vi "CRY6181 Run Seq.vi"() -> ()   [LabVIEW 2013]
uses:
  CRYSystem/Typedef Control/CRYData Cluster.ctl
  CRYSystem/Typedef Control/CRYResult Cluster.ctl
  CRYSystem/Typedef Control/CRYWaveform Cluster.ctl
  CRYWindow/SubVI/CRYMain Sub Window Global.vi
  CRYProject/CRYProject Editor Global.vi
  CRYMainGlobal.vi
  CRYSystem/Task Sequence/CRYProject Run Control Global.vi
panel:
  in  "Tab Control":enum32{"Parameter", "Data"}(tab)
  out "Margin":dbl
  out "Duration":dbl
  out "Passed?":bool
  out "Ran to completion":bool
  in  "path":path caption="Sequence to run (full path)"
  in  "Serial #":string
  in  "Lot #":string
  in  "Mode":enum16{"Load Sequence", "Run Sequence", "All"}(ring)
  out "Data Array":T1[](array[typedef]) {"Z data" items=["dB", "Lin"]; "X data" items=["dB", "Lin"]; "Y data" items=["dB", "Lin"]; "Z dB ref" format="%.1f"; "Z axis" items=["Log", "Lin"]; "X dB ref" format="%.1f"; "X axis" items=["Log", "Lin"]; "Y axis" items=["Log", "Lin"]; "Y dB ref" format="%.1f"; "Curve"."z" format="%.2f"; "Curve"."y" format="%.2f"; "Curve"."x" format="%.2f"}
  out "Results Array":T2[](array[typedef]) {"Margin" format="%.2f"}
  out "Waveforms Array":T3[](array[typedef]) {"Y dB ref" format="%.1f"; "Y axis" items=["Log", "Lin"]; "Y data" items=["dB", "Lin"]; "X data" items=["dB", "Lin"]}
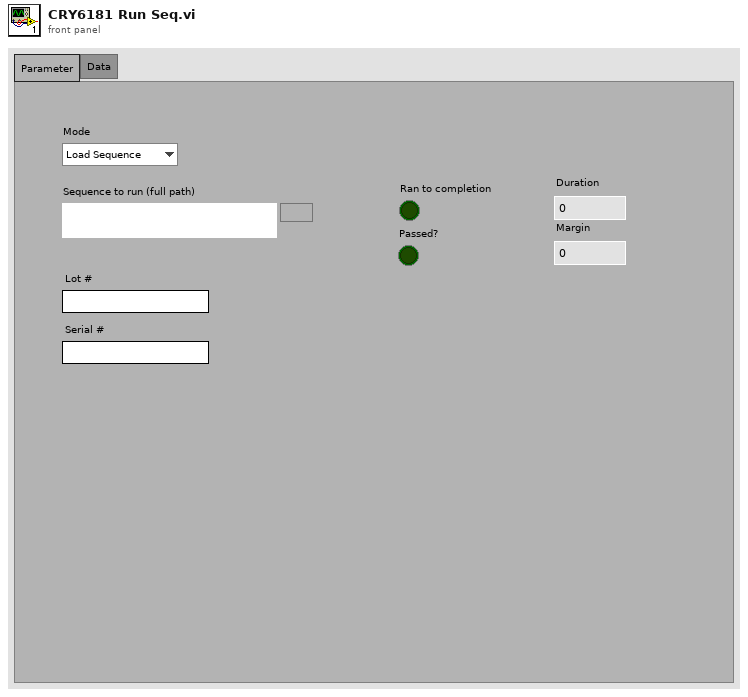
[diagram p1: front panel]
types:
  T1 = typedef "CRYData Cluster.ctl" = cluster{"Name":string, "Curve":cluster{"x":dbl, "y":dbl, "z":dbl}[], "X data":u16, "Y data":u16, "Z data":u16, "X axis":u16, "Y axis":u16, "Z axis":u16, "X unit":string, "Y unit":string, "Z unit":string, "X dB ref":dbl, "Y dB ref":dbl, "Z dB ref":dbl, "single val":bool, "protected":bool, "display X":bool, "display Y":bool, "display Z":bool, "Test Info":string, "Step No.":i32, "Plot Settings":cluster{"Color":u32, "Interpolation":u8, "Point Style":u8, "Line Style":u8, "Point Color":u32, "Line Width":u8, "Bar Plot Style":u8, "Fill To":i16}, "AutoProtect":bool}
  T2 = typedef "CRYResult Cluster.ctl" = cluster{"Name":string, "Margin":dbl, "unit":string, "Verdict":bool, "Limit":string, "Max/Min":string, "protected":bool, "Step No.":i32, "Test Info":string, "AutoProtect":bool}
  T3 = typedef "CRYWaveform Cluster.ctl" = cluster{"Waveform":cluster{"X0":dbl, "dX":dbl, "Y":sgl[]}, "X data":u16, "Y data":u16, "Y axis":u16, "X unit":string, "Y unit":string, "Y dB ref":dbl, "display Y":bool, "display X":bool, "Overload?":bool, "Test Info":string, "Step No.":i32, "Name":string, "protected":bool, "Sqc history":string[], "Signal Channel ID":i32, "Plot Settings":cluster{"Color":u32, "Interpolation":u8, "Point Style":u8, "Line Style":u8, "Point Color":u32, "Line Width":u8, "Bar Plot Style":u8, "Fill To":i16}, "AutoProtect":bool}
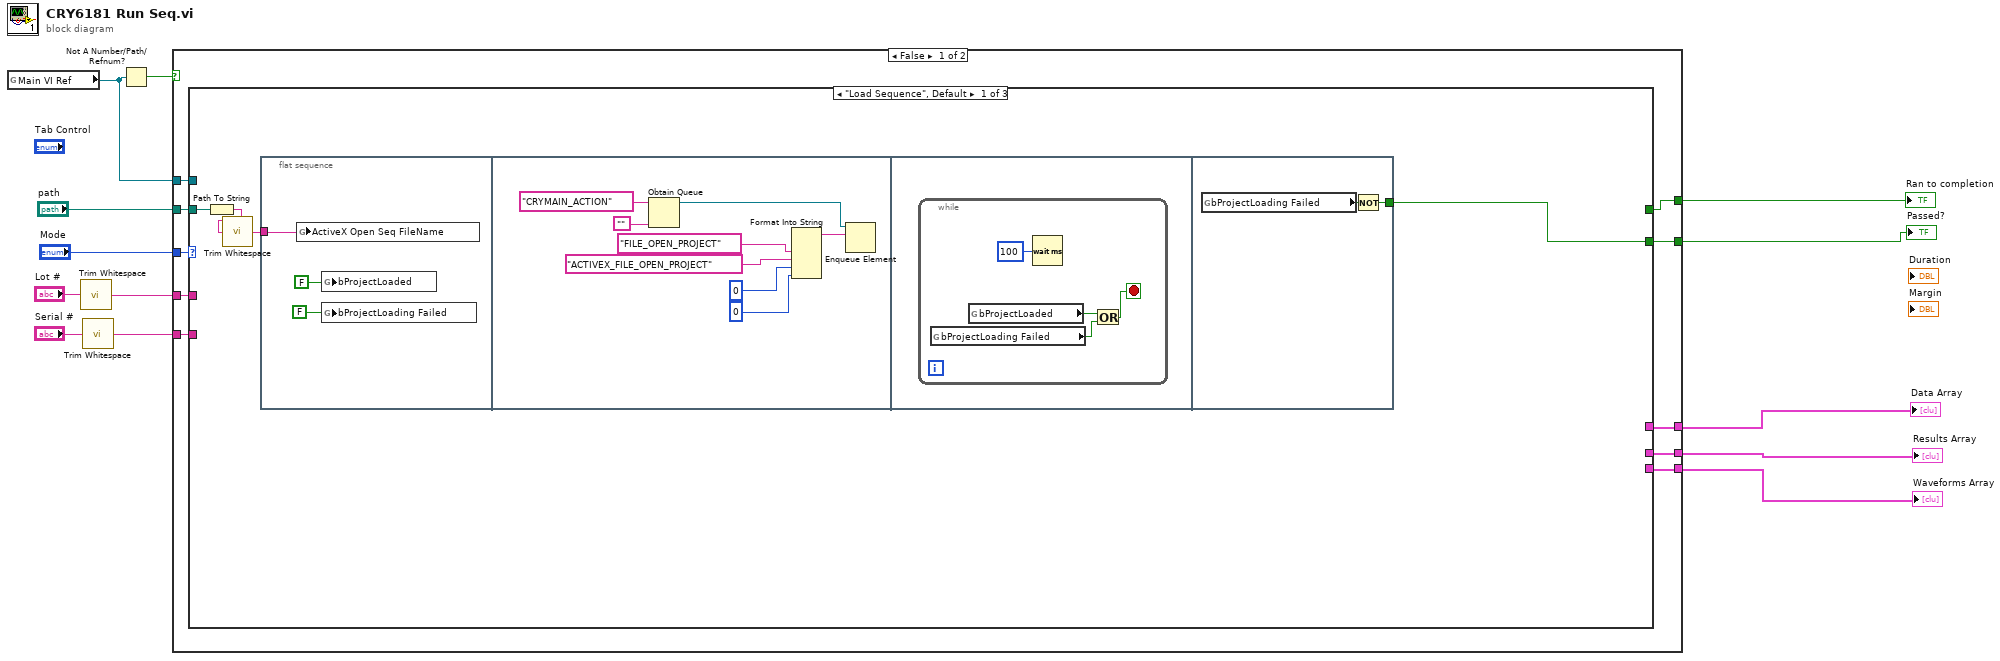
[diagram p0: block diagram]
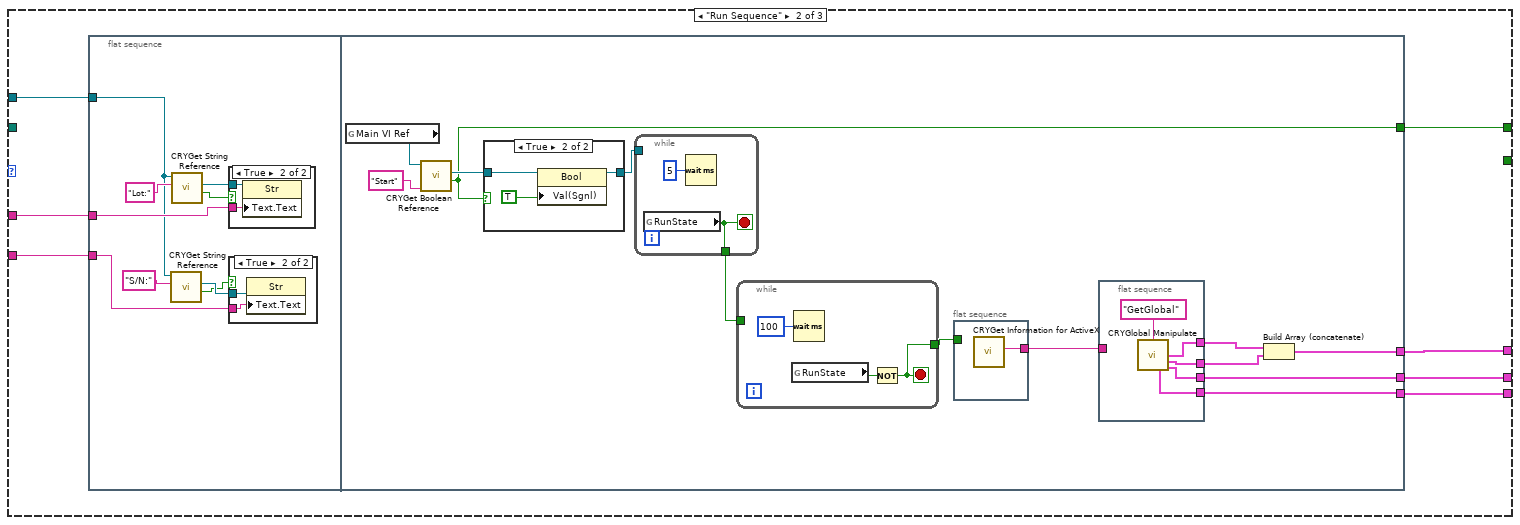
[diagram p2: hidden frame]
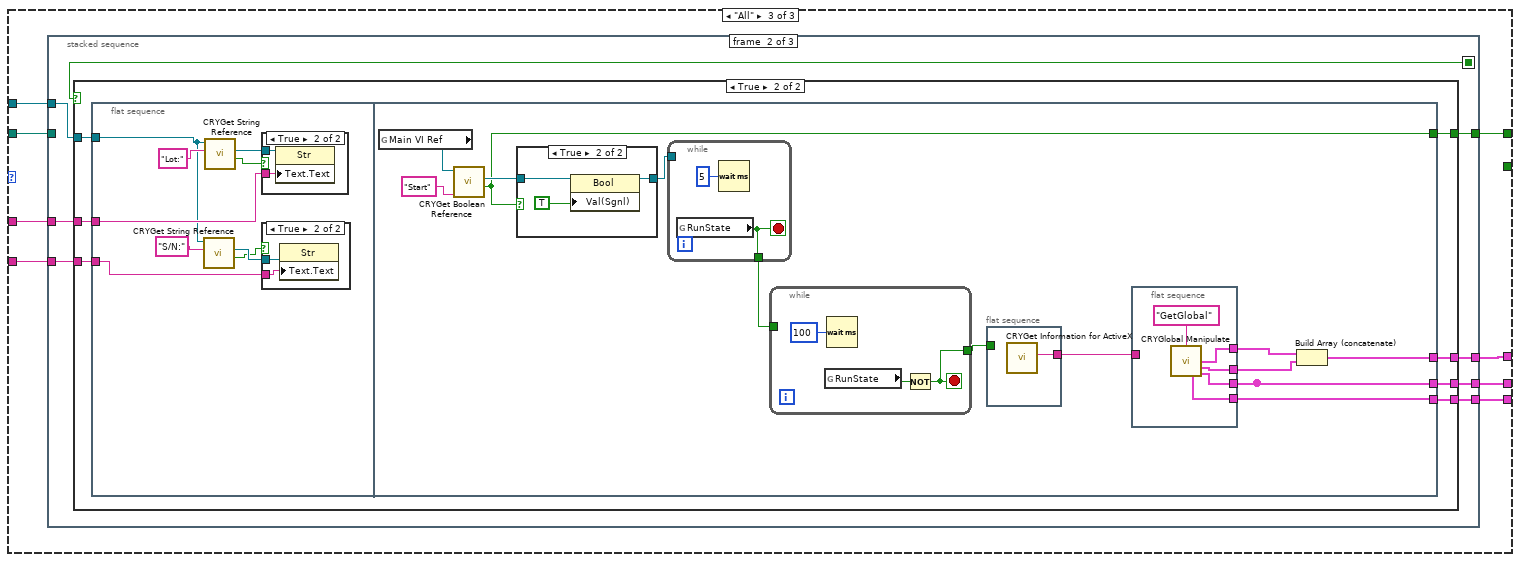
[diagram p6: hidden frame]
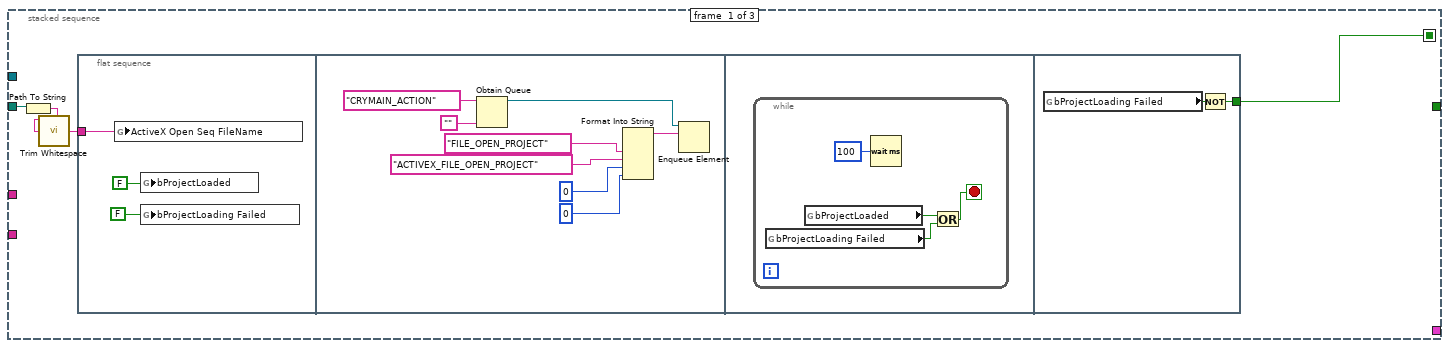
[diagram p7: hidden frame]
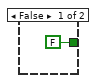
[diagram p8: hidden frame]
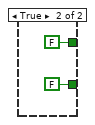
[diagram p13: hidden frame]
diagram:
  n1 = global read "CRYMain Sub Window Global.vi" "Main VI Ref"() -> (w1:refnum<vi>)
  n2 = call <vilib>:"Trim Whitespace.vi"("string"="Lot #") -> ("trimmed string"=w11:string)  [unwired: 1 in]
  n3 = call <vilib>:"Trim Whitespace.vi"("string"="Serial #") -> ("trimmed string"=w9:string)  [unwired: 1 in]
  n4 = Not A Number/Path/Refnum?(number/path/refnum=w1) -> (NaN/Path/Refnum?=w2:bool)
  n5 = case shown="False" w2 {
    tunnel: "Mode" -> [w23 _]
    tunnel: w11 -> [w22 _]
    tunnel: w9 -> [w21 _]
    tunnel: [w20 FALSE ("Exist?")] -> w8
    tunnel: [w19 _] -> w7
    tunnel: [w18 _] -> w6
    tunnel: [w17 _] -> w5
    tunnel: "path" -> [w16 _]
    tunnel: [w15 FALSE] -> w3
    tunnel: w1 -> [w14 _]
    frame False {
      n6 = case shown="\"Load Sequence\", Default" w23 {
        tunnel: w22 -> [_ w51 w99]
        tunnel: w21 -> [_ w50 w98]
        tunnel: [_ w49 w94] -> w20
        tunnel: [_ w48 w97] -> w19
        tunnel: [_ w47 w96] -> w18
        tunnel: [_ w46 w95] -> w17
        tunnel: w16 -> [w27 _ w100]
        tunnel: [w24 _ _] -> w15
        tunnel: w14 -> [_ w45 w93]
        frame "Load Sequence", Default {
          n7 = Path To String(path=w27) -> (string=w25:string)
          n8 = call <vilib>:"Trim Whitespace.vi"("string"=w25) -> ("trimmed string"=w26:string)  [unwired: 1 in]
          n9 = flat-sequence {
            tunnel: w26 -> [w30]
            tunnel: [w43] -> w24
            frame #0 {
              n10 = global write "CRYMainGlobal.vi" "ActiveX Open Seq FileName"(w30) -> ()
              n11 = global write "CRYProject Editor Global.vi" "bProjectLoaded"(FALSE (".not. x?")) -> ()
              n12 = global write "CRYProject Editor Global.vi" "bProjectLoading Failed"(FALSE ("bProjectLoaded Failed")) -> ()
            }
            frame #1 {
              n13 = Obtain Queue(name (unnamed)="CRYMAIN_ACTION" ("YAxisTitle"), element data type="" ("Action Type")) -> (queue out=w32:refnum<queue>)  [unwired: 3 in, 2 out]
              n14 = Format Into String("FILE_OPEN_PROJECT" ("input 1"), "ACTIVEX_FILE_OPEN_PROJECT" ("input 2"), 0 ("input 2"), 0 ("input 3")) -> (resulting string=w37:string)  [unwired: 3 in, 1 out]
              n15 = Enqueue Element(queue=w32, element=w37) -> ()  [unwired: 1 in, 4 out]
            }
            frame #2 {
              n16 = while {
                stop <- w39 stop-if-true
                n17 = global read "CRYProject Editor Global.vi" "bProjectLoading Failed"() -> (w40:bool)
                n18 = global read "CRYProject Editor Global.vi" "bProjectLoaded"() -> (w41:bool)
                n19 = Wait (ms)(milliseconds to wait=u32 100) -> ()  [unwired: 1 out]
                n20 = Or(x=w41, y=w40) -> (x .or. y?=w39:bool)
              }
            }
            frame #3 {
              n21 = global read "CRYProject Editor Global.vi" "bProjectLoading Failed"() -> (w44:bool)
              n22 = Not(x=w44) -> (.not. x?=w43:bool)
            }
          }
        }
        frame "Run Sequence" {
          n23 = flat-sequence {
            tunnel: w51 -> [w57]
            tunnel: w50 -> [w54]
            tunnel: w45 -> [w52]
            tunnel: [w71] -> w49
            tunnel: [w67] -> w48
            tunnel: [w66] -> w46
            tunnel: [w65] -> w47
            frame #0 {
              n24 = call "CRYGet String Reference.vi"("Label Name"="S/N:", "VI Refnum"=w52) -> ("Find?"=w53:bool, "String Ref Out"=w55:refnum<vi>)  [unwired: 7 in, 1 out]
              n25 = call "CRYGet String Reference.vi"("Label Name"="Lot:", "VI Refnum"=w52) -> ("Find?"=w58:bool, "String Ref Out"=w59:refnum<vi>)  [unwired: 7 in, 1 out]
              n26 = case shown="True" w58 {
                tunnel: w59 -> [_ w64]
                tunnel: w57 -> [_ w63]
                frame False {
                }
                frame True {
                  n27 = property class="Str"(reference=w64, "Text.Text"=w63) -> ()  [unwired: 1 in, 2 out]
                }
              }
              n28 = case shown="True" w53 {
                tunnel: w55 -> [_ w62]
                tunnel: w54 -> [_ w61]
                frame False {
                }
                frame True {
                  n29 = property class="Str"(reference=w62, "Text.Text"=w61) -> ()  [unwired: 1 in, 2 out]
                }
              }
            }
            frame #1 {
              n30 = global read "CRYMain Sub Window Global.vi" "Main VI Ref"() -> (w72:refnum<vi>)
              n31 = call "CRYGet Boolean Reference.vi"("Label Name"="Start", "VI Refnum"=w72) -> ("Exist?"=w71:bool, "Boolean Ref"=w74:refnum<vi>)  [unwired: 7 in, 1 out]
              n32 = case shown="True" w71 {
                tunnel: w74 -> [w89 w92]
                tunnel: [w89 w90] -> w76
                frame False {
                }
                frame True {
                  n33 = property class="Bool"(reference=w92, "Val(Sgnl)"=TRUE ("Boolean")) -> (reference out=w90:refnum<vi>)  [unwired: 1 in, 1 out]
                }
              }
              n34 = while {
                tunnel: [w83] -> w77
                tunnel: w76 -> [_]
                stop <- w83 stop-if-true
                n35 = global read "CRYProject Run Control Global.vi" "RunState"() -> (w83:bool)
                n36 = Wait (ms)(milliseconds to wait=u32 5) -> ()  [unwired: 1 out]
              }
              n37 = while {
                tunnel: [w86] -> w75
                tunnel: w77 -> [_]
                stop <- w86 stop-if-true
                n38 = global read "CRYProject Run Control Global.vi" "RunState"() -> (w88:bool)
                n39 = Wait (ms)(milliseconds to wait=u32 100) -> ()  [unwired: 1 out]
                n40 = Not(x=w88) -> (.not. x?=w86:bool)
              }
              n41 = flat-sequence {
                tunnel: [w85] -> w70
                tunnel: w75 -> [_]
                frame #0 {
                  n42 = call "CRYGet Information for ActiveX.vi"() -> ("Limit Array Out"=w85:string)  [unwired: 10 in, 1 out]
                }
              }
              n43 = flat-sequence {
                tunnel: w70 -> [_]
                tunnel: [w81] -> w69
                tunnel: [w80] -> w68
                tunnel: [w79] -> w65
                tunnel: [w78] -> w66
                frame #0 {
                  n44 = call "CRYGlobal Manipulate.vi"("sAction"="GetGlobal") -> ("Curves Out"=w81:T1[], "Values Out"=w80:T1[], "WFM Out"=w78:T3[], "Results Out"=w79:T2[])  [unwired: 8 in, 3 out]
                }
              }
              n45 = Build Array (concatenate)(w69, w68) -> (w67:T1[])
            }
          }
        }
        frame "All" {
          n46 = stacked-sequence {
            seq-local: [w101 _ _] -> [_ w127 _]
            tunnel: w100 -> [w102 _ _]
            tunnel: w99 -> [_ w129 _]
            tunnel: w98 -> [_ w128 _]
            tunnel: [_ w126 _] -> w97
            tunnel: [_ w125 _] -> w96
            tunnel: [_ w124 _] -> w95
            tunnel: [_ w123 _] -> w94
            tunnel: w93 -> [_ w122 _]
            frame #0 {
              n47 = Path To String(path=w102) -> (string=w103:string)
              n48 = call <vilib>:"Trim Whitespace.vi"("string"=w103) -> ("trimmed string"=w104:string)  [unwired: 1 in]
              n49 = flat-sequence {
                tunnel: w104 -> [w107]
                tunnel: [w120] -> w101
                frame #0 {
                  n50 = global write "CRYMainGlobal.vi" "ActiveX Open Seq FileName"(w107) -> ()
                  n51 = global write "CRYProject Editor Global.vi" "bProjectLoaded"(FALSE (".not. x?")) -> ()
                  n52 = global write "CRYProject Editor Global.vi" "bProjectLoading Failed"(FALSE ("bProjectLoaded Failed")) -> ()
                }
                frame #1 {
                  n53 = Obtain Queue(name (unnamed)="CRYMAIN_ACTION" ("YAxisTitle"), element data type="" ("Action Type")) -> (queue out=w109:refnum<queue>)  [unwired: 3 in, 2 out]
                  n54 = Format Into String("FILE_OPEN_PROJECT" ("input 1"), "ACTIVEX_FILE_OPEN_PROJECT" ("input 2"), 0 ("input 2"), 0 ("input 3")) -> (resulting string=w114:string)  [unwired: 3 in, 1 out]
                  n55 = Enqueue Element(queue=w109, element=w114) -> ()  [unwired: 1 in, 4 out]
                }
                frame #2 {
                  n56 = while {
                    stop <- w116 stop-if-true
                    n57 = global read "CRYProject Editor Global.vi" "bProjectLoading Failed"() -> (w117:bool)
                    n58 = global read "CRYProject Editor Global.vi" "bProjectLoaded"() -> (w118:bool)
                    n59 = Wait (ms)(milliseconds to wait=u32 100) -> ()  [unwired: 1 out]
                    n60 = Or(x=w118, y=w117) -> (x .or. y?=w116:bool)
                  }
                }
                frame #3 {
                  n61 = global read "CRYProject Editor Global.vi" "bProjectLoading Failed"() -> (w121:bool)
                  n62 = Not(x=w121) -> (.not. x?=w120:bool)
                }
              }
            }
            frame #1 {
              n63 = case shown="True" w127 {
                tunnel: w129 -> [_ w137]
                tunnel: w128 -> [_ w136]
                tunnel: [_ w135] -> w126
                tunnel: [_ w134] -> w125
                tunnel: [_ w133] -> w124
                tunnel: [FALSE ("Exist?") w132] -> w123
                tunnel: w122 -> [_ w131]
                frame False {
                }
                frame True {
                  n64 = flat-sequence {
                    tunnel: w137 -> [w143]
                    tunnel: w136 -> [w140]
                    tunnel: w131 -> [w138]
                    tunnel: [w157] -> w132
                    tunnel: [w153] -> w135
                    tunnel: [w152] -> w133
                    tunnel: [w151] -> _
                    tunnel: [w151] -> w134
                    frame #0 {
                      n65 = call "CRYGet String Reference.vi"("Label Name"="S/N:", "VI Refnum"=w138) -> ("Find?"=w139:bool, "String Ref Out"=w141:refnum<vi>)  [unwired: 7 in, 1 out]
                      n66 = call "CRYGet String Reference.vi"("Label Name"="Lot:", "VI Refnum"=w138) -> ("Find?"=w144:bool, "String Ref Out"=w145:refnum<vi>)  [unwired: 7 in, 1 out]
                      n67 = case shown="True" w144 {
                        tunnel: w145 -> [_ w150]
                        tunnel: w143 -> [_ w149]
                        frame False {
                        }
                        frame True {
                          n68 = property class="Str"(reference=w150, "Text.Text"=w149) -> ()  [unwired: 1 in, 2 out]
                        }
                      }
                      n69 = case shown="True" w139 {
                        tunnel: w141 -> [_ w148]
                        tunnel: w140 -> [_ w147]
                        frame False {
                        }
                        frame True {
                          n70 = property class="Str"(reference=w148, "Text.Text"=w147) -> ()  [unwired: 1 in, 2 out]
                        }
                      }
                    }
                    frame #1 {
                      n71 = global read "CRYMain Sub Window Global.vi" "Main VI Ref"() -> (w158:refnum<vi>)
                      n72 = call "CRYGet Boolean Reference.vi"("Label Name"="Start", "VI Refnum"=w158) -> ("Exist?"=w157:bool, "Boolean Ref"=w160:refnum<vi>)  [unwired: 7 in, 1 out]
                      n73 = case shown="True" w157 {
                        tunnel: w160 -> [w175 w178]
                        tunnel: [w175 w176] -> w162
                        frame False {
                        }
                        frame True {
                          n74 = property class="Bool"(reference=w178, "Val(Sgnl)"=TRUE ("Boolean")) -> (reference out=w176:refnum<vi>)  [unwired: 1 in, 1 out]
                        }
                      }
                      n75 = while {
                        tunnel: [w169] -> w163
                        tunnel: w162 -> [_]
                        stop <- w169 stop-if-true
                        n76 = global read "CRYProject Run Control Global.vi" "RunState"() -> (w169:bool)
                        n77 = Wait (ms)(milliseconds to wait=u32 5) -> ()  [unwired: 1 out]
                      }
                      n78 = while {
                        tunnel: [w172] -> w161
                        tunnel: w163 -> [_]
                        stop <- w172 stop-if-true
                        n79 = global read "CRYProject Run Control Global.vi" "RunState"() -> (w174:bool)
                        n80 = Wait (ms)(milliseconds to wait=u32 100) -> ()  [unwired: 1 out]
                        n81 = Not(x=w174) -> (.not. x?=w172:bool)
                      }
                      n82 = flat-sequence {
                        tunnel: [w171] -> w156
                        tunnel: w161 -> [_]
                        frame #0 {
                          n83 = call "CRYGet Information for ActiveX.vi"() -> ("Limit Array Out"=w171:string)  [unwired: 10 in, 1 out]
                        }
                      }
                      n84 = flat-sequence {
                        tunnel: w156 -> [_]
                        tunnel: [w167] -> w155
                        tunnel: [w166] -> w154
                        tunnel: [w165] -> w151
                        tunnel: [w164] -> w152
                        frame #0 {
                          n85 = call "CRYGlobal Manipulate.vi"("sAction"="GetGlobal") -> ("Curves Out"=w167:T1[], "Values Out"=w166:T1[], "WFM Out"=w164:T3[], "Results Out"=w165:T2[])  [unwired: 8 in, 3 out]
                        }
                      }
                      n86 = Build Array (concatenate)(w155, w154) -> (w153:T1[])
                    }
                  }
                }
              }
            }
            frame #2 {
            }
          }
        }
      }
    }
    frame True {
    }
  }
  "Ran to completion" <- w8
  "Passed?" <- w3
  "Data Array" <- w7
  "Results Array" <- w6
  "Waveforms Array" <- w5
